vi "SubVI_Res-ch_add.vi"(7 "cmd":enum16{"ini", "Res add", "read"}(ring), 8 "error in (no error)":errorcluster caption="에러 입력(에러 없음)", 11 "Resister data":T1) -> (0 "error out":errorcluster caption="에러 출력", 3 "Result Table update":T2)   [LabVIEW 2016]
uses:
  Ctrls/raw data type.ctl
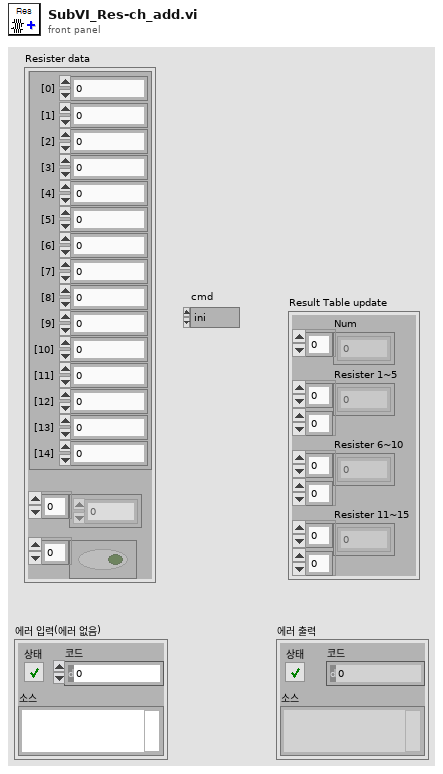
[diagram p1: front panel]
types:
  T1 = typedef "raw data type.ctl" = cluster{"Resistor values":cluster{"[0]":dbl, "[1]":dbl, "[2]":dbl, "[3]":dbl, "[4]":dbl, "[5]":dbl, "[6]":dbl, "[7]":dbl, "[8]":dbl, "[9]":dbl, "[10]":dbl, "[11]":dbl, "[12]":dbl, "[13]":dbl, "[14]":dbl}, "Resistor tables":u8[], "Pass Fails":bool[]}
  T2 = cluster{"Num":u32[], "Resister 1~5":u8[][], "Resister 6~10":u8[][], "Resister 11~15":u8[][]}
  T3 = typedef "Total data.ctl" = cluster{"Raw Data":T4, "Resister result data":T1, "Result Table update":cluster{"Num":u32[], "Resister 1~5":u8[][], "Resister 6~10":u8[][], "Resister 11~15":u8[][]}, "Strain Data":cluster{"Strain 1":dbl, "Strain 2":dbl, "Strain 3":dbl, "Strain 4":dbl}, "Acc Result":cluster{"Acc Peak":dbl, "Acc time":dbl, "Acc area":dbl}, "STATUS":cluster{"status":string, "all_fail":bool, "emg":bool, "cycle":u16, "file name":string}, "Speed":dbl, "Acc peak time":dbl, "Max Strain":dbl, "Resistor at peak":cluster{"[0]":dbl, "[1]":dbl, "[2]":dbl, "[3]":dbl, "[4]":dbl, "[5]":dbl, "[6]":dbl, "[7]":dbl, "[8]":dbl, "[9]":dbl, "[10]":dbl, "[11]":dbl, "[12]":dbl, "[13]":dbl, "[14]":dbl}, "Acc peak index":u32, "time":string, "Cycle finish":bool, "Resistor at ini":cluster{"[0]":dbl, "[1]":dbl, "[2]":dbl, "[3]":dbl, "[4]":dbl, "[5]":dbl, "[6]":dbl, "[7]":dbl, "[8]":dbl, "[9]":dbl, "[10]":dbl, "[11]":dbl, "[12]":dbl, "[13]":dbl, "[14]":dbl}}
  T4 = typedef "raw Q data.ctl" = cluster{"Res_data":waveform(dbl)[], "Acc_data":waveform(dbl), "Strain_data":waveform(dbl)[]}
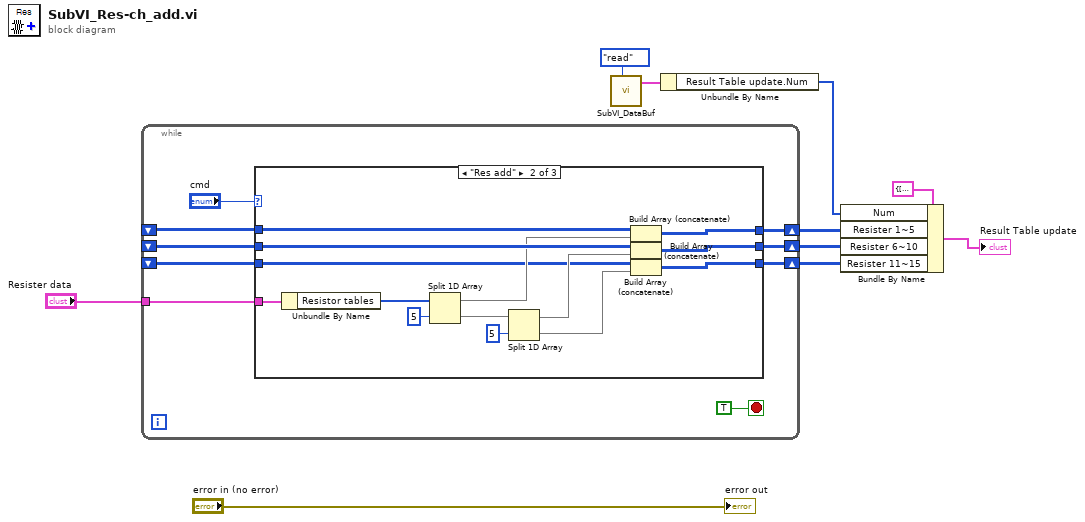
[diagram p0: block diagram]
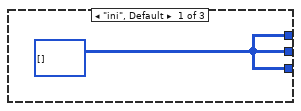
[diagram p2: hidden frame]
diagram:
  n1 = while {
    shift-right: [w17] -> w6
    shift-left: _ -> [w16]
    shift-right: [w15] -> w7
    shift-left: _ -> [w12]
    shift-right: [w14] -> w8
    shift-left: _ -> [w13]
    tunnel: "Resister data" -> [w11]
    stop <- TRUE stop-if-true
    n2 = case shown="\"Res add\"" "cmd" {
      tunnel: [w20 w23 w37] -> w17
      tunnel: w16 -> [_ w25 w37]
      tunnel: [w20 w24 w36] -> w15
      tunnel: [w20 w30 w35] -> w14
      tunnel: w13 -> [_ w31 w35]
      tunnel: w12 -> [_ w29 w36]
      tunnel: w11 -> [_ w21 _]
      frame "ini", Default {
        w20 = u8[][] [] ("Result Table data")
      }
      frame "Res add" {
        n3 = Unbundle By Name(w21) -> ("Resistor tables"=w22:u8[])
        n4 = Split 1D Array(array=w22, index=5 ("인덱스")) -> (first subarray=w28:u8[], second subarray=w34:u8[])
        n5 = Split 1D Array(array=w34, index=5 ("인덱스")) -> (first subarray=w27:u8[], second subarray=w26:u8[])
        n6 = Build Array (concatenate)(w31, w28) -> (w30:u8[][])
        n7 = Build Array (concatenate)(w29, w27) -> (w24:u8[][])
        n8 = Build Array (concatenate)(w25, w26) -> (w23:u8[][])
      }
      frame "read" {
      }
    }
  }
  n9 = call "SubVI_DataBuf.vi"("cmd"=enum16{"ini", "write", "read"}."read") -> ("Total data 2"=w2:T3)  [unwired: 9 in, 1 out]
  n10 = Unbundle By Name(w2) -> ("Result Table update.Num"=w1:u32[])
  n11 = Bundle By Name(cluster=T2 {"Num"=[1, 2, 3, 4, 5, 6, 7, 8, 9, 10, 11, 12, 13, 14, 15, 16, 17, 18, 19, 20, 21, 22, 23, 24, 25, 26, 27, 28, 29, 30, 31, 32, 33, 34, 35, 36, 37, 38, 39, 40, 41, 42, 43, 44, 45, 46, 47, 48, 49, 50, 51, 52, 53, 54, 55, 56, 57, 58, 59, 60, 61, 62, 63, 64, 65, 66, 67, 68, 69, 70, 71, 72, 73, 74, 75, 76, 77, 78, 79, 80, 81, 82, 83, 84, 85, 86, 87, 88, 89, 90, 91, 92, 93, 94, 95, 96, 97, 98, 99, 100], "Resister 1~5"=[[1, 1, 1, 0, 0], [1, 1, 1, 0, 0], [1, 1, 1, 0, 0], [1, 1, 1, 0, 0], [1, 1, 1, 0, 0], [1, 1, 1, 0, 0], [1, 1, 1, 0, 0], [1, 1, 1, 0, 0], [1, 1, 1, 0, 0], [1, 1, 1, 0, 0]], "Resister 6~10"=[[1, 1, 1, 1, 0], [1, 1, 1, 1, 0], [1, 1, 1, 1, 0], [1, 1, 1, 1, 0], [1, 1, 1, 1, 0], [1, 1, 1, 1, 0], [1, 1, 1, 1, 0], [1, 1, 1, 1, 0], [1, 1, 1, 1, 0], [1, 1, 1, 1, 0]], "Resister 11~15"=[[0, 0, 1, 1, 1], [0, 0, 1, 1, 1], [0, 0, 1, 1, 1], [0, 0, 1, 1, 1], [0, 0, 1, 1, 1], [0, 0, 1, 1, 1], [0, 0, 1, 1, 1], [0, 0, 1, 1, 1], [0, 0, 1, 1, 1], [0, 0, 1, 1, 1]]} ("Result Table"), "Num"=w1, "Resister 1~5"=w8, "Resister 6~10"=w7, "Resister 11~15"=w6) -> (→"Result Table update":T2)
  "error out" <- "error in (no error)"
